vi "calc CG.vi"(8 "error in (no error)":errorcluster) -> (0 "error out":errorcluster)   [LabVIEW 2023]
uses:
  ctrl defs/ctrl swerve module.ctl
  ctrl defs/ctrl XY coord.ctl
  Global INIT.vi
  Global odometry.vi
panel:
  out "SWERVE INFO written to Global  odometry file":T1[](array[typedef]) {"corner wt (lbm)" format="%#.3f"; "POS" format="%.3g"; "coord wrt geom CTR"."geomY" format="%.4g"; "coord wrt geom CTR"."geomX" format="%.4g"; "from pivot to module"."theta spin (deg)" format="%.4g"; "from pivot to module"."theta (deg)" format="%.4g"; "from pivot to module"."R" format="%.4g"; "ABS" format="%.3g"; "target" format="%.3g"; "V" format="%.3g"}
  out "coord wrt geom ctr":cluster{"X":dbl, "Y":dbl}[](array[cluster])
  out "CG XY":cluster{"X":dbl, "Y":dbl}
  out "wheel track & base":cluster{"X":dbl, "Y":dbl}={"X"=24.428, "Y"=24.428}
  out "weight (lbm)":dbl
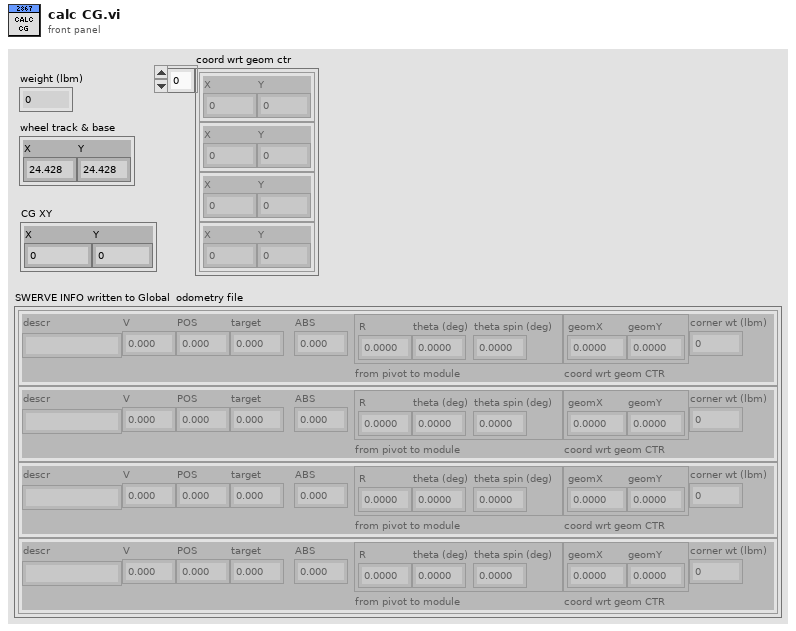
[diagram p1: front panel]
types:
  T1 = typedef "ctrl swerve module.ctl" = cluster{"descr":string, "V":dbl, "POS":dbl, "target":dbl, "ABS":dbl, "from pivot to module":cluster{"R":dbl, "theta (deg)":dbl, "theta spin (deg)":dbl}, "coord wrt geom CTR":cluster{"geomX":dbl, "geomY":dbl}, "corner wt (lbm)":dbl}
  T2 = typedef "ctrl XY coord.ctl" = cluster{"X":dbl, "Y":dbl}
  T3 = typedef "ctrl robot swerve dims.ctl" = cluster{"drive track":dbl, "drive base":dbl, "wheel  (in)":dbl, "steer ratio":dbl, "drive ratio":dbl, "enc ratio":dbl}
  T4 = cluster{"description":string, "wrt geom CTR":cluster{"delX":i8, "delY":i8}}[]
  T5 = typedef "ctrl robot CG.ctl" = cluster{"mass (lbm)":dbl, "CG":T2, "Zcg":dbl}
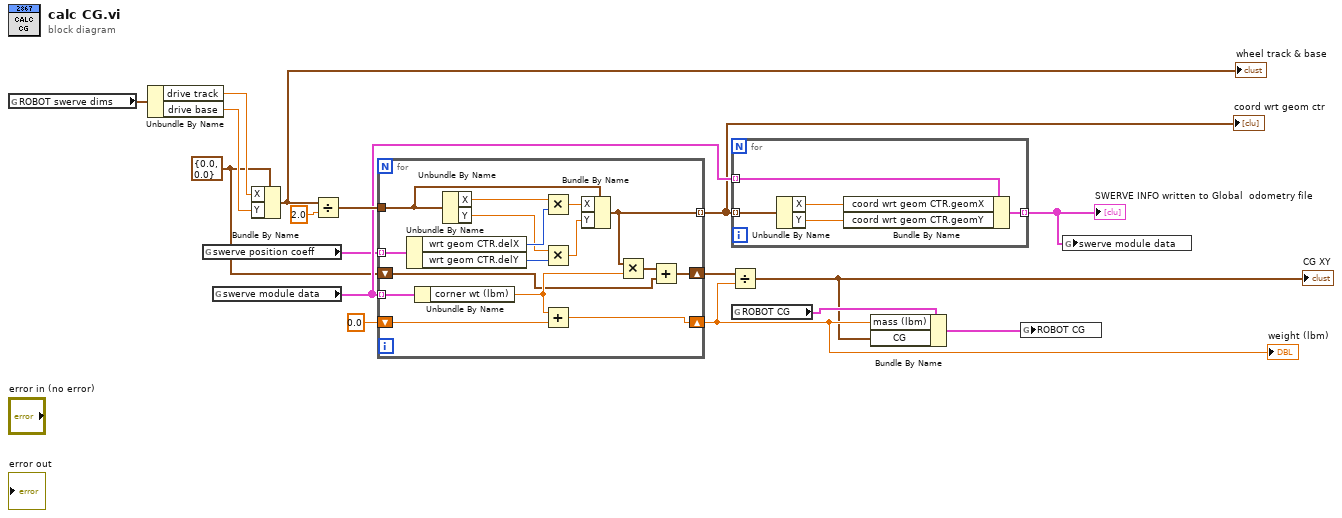
[diagram p0: block diagram]
diagram:
  w2 = T2 {"X"=0.0, "Y"=0.0} ("pivot center")
  n1 = global read "Global INIT.vi" "ROBOT swerve dims"() -> (w11:T3)
  n2 = Unbundle By Name(w11) -> ("drive track"=w15:dbl, "drive base"=w14:dbl)
  n3 = global read "Global INIT.vi" "swerve position coeff"() -> (w1:T4)
  n4 = global read "Global odometry.vi" "swerve module data"() -> (w6:T1[])
  n5 = Bundle By Name(cluster=w2, "X"=w15, "Y"=w14) -> (w13:T2)
  "wheel track & base" <- w13
  n6 = Divide(x=w13, y=2.0) -> (x/y=w10:T2)
  n7 = for {
    tunnel: w10 -> [w33]
    tunnel: [w24] -> w4 mode=indexing
    tunnel: w6 -> [w30] mode=indexing
    shift-right: [w23] -> w8
    shift-left: 0.0 -> [w29]
    shift-right: [w20] -> w7
    shift-left: w2 -> [w19]
    tunnel: w1 -> [w18] mode=indexing
    n8 = Unbundle By Name(w18) -> ("wrt geom CTR.delX"=w28:i8, "wrt geom CTR.delY"=w25:i8)
    n9 = Unbundle By Name(w30) -> ("corner wt (lbm)"=w22:dbl)
    n10 = Unbundle By Name(w33) -> ("X"=w31:dbl, "Y"=w26:dbl)
    n11 = Multiply(x=w31, y=w28) -> (x*y=w32:dbl)
    n12 = Multiply(x=w26, y=w25) -> (x*y=w27:dbl)
    n13 = Add(x=w22, y=w29) -> (x+y=w23:dbl)
    n14 = Bundle By Name(cluster=w33, "X"=w32, "Y"=w27) -> (w24:T2)
    n15 = Multiply(x=w24, y=w22) -> (x*y=w21:T2)
    n16 = Add(x=w21, y=w19) -> (x+y=w20:T2)
  }
  "weight (lbm)" <- w8
  "coord wrt geom ctr" <- w4
  n17 = Divide(x=w7, y=w8) -> (x/y=w3:T2)
  "CG XY" <- w3
  n18 = for {
    tunnel: w6 -> [w38] mode=indexing
    tunnel: [w37] -> w5 mode=indexing
    tunnel: w4 -> [w36] mode=indexing
    n19 = Unbundle By Name(w36) -> ("X"=w35:dbl, "Y"=w34:dbl)
    n20 = Bundle By Name(cluster=w38, "coord wrt geom CTR.geomX"=w35, "coord wrt geom CTR.geomY"=w34) -> (w37:T1)
  }
  "SWERVE INFO written to Global  odometry file" <- w5
  n21 = global read "Global INIT.vi" "ROBOT CG"() -> (w17:T5)
  n22 = Bundle By Name(cluster=w17, "mass (lbm)"=w8, "CG"=w3) -> (w16:T5)
  n23 = global write "Global INIT.vi" "ROBOT CG"(w16) -> ()
  n24 = global write "Global odometry.vi" "swerve module data"(w5) -> ()
